vi "Unflatten.vi"(8 "error in (no error)":errorcluster, 11 "LCD Reader in":refnum<class "LCD Reader.lvclass">) -> (0 "error out":errorcluster, 3 "LCD Reader out":refnum<class "LCD Reader.lvclass">)   [LabVIEW 2012, in "LCD Reader.lvclass"]
uses:
  LCD Reader.lvclass
  Reader/Reader.lvclass
  LCD Reader.lvclass/LCD Reader.ctl
  Global/File Locations.vi
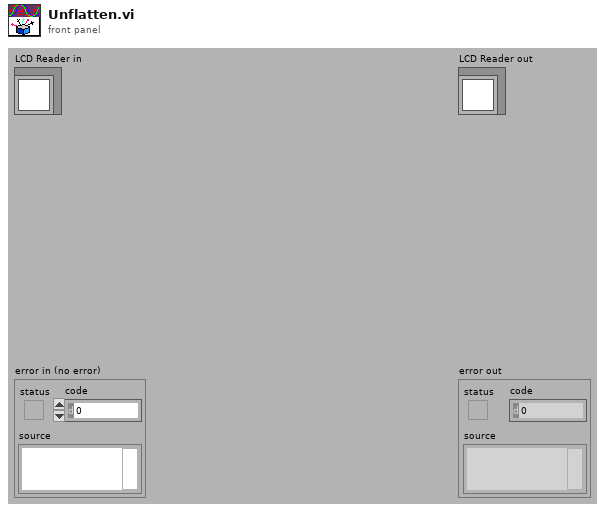
[diagram p1: front panel]
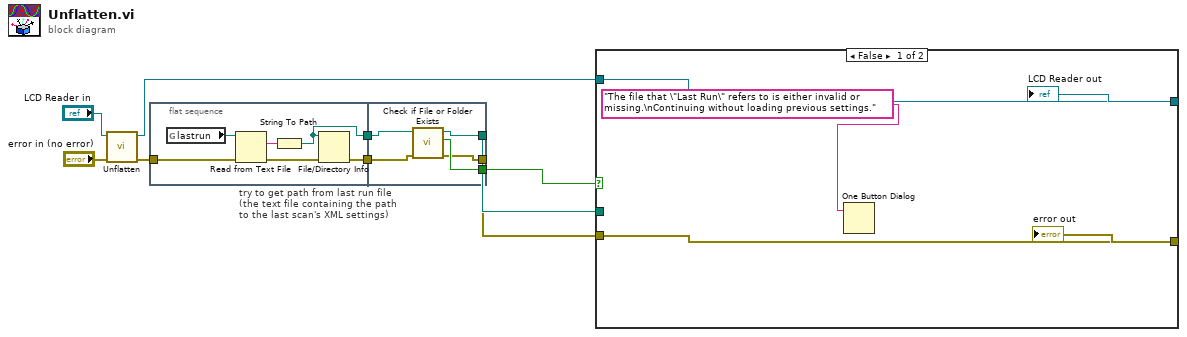
[diagram p0: block diagram]
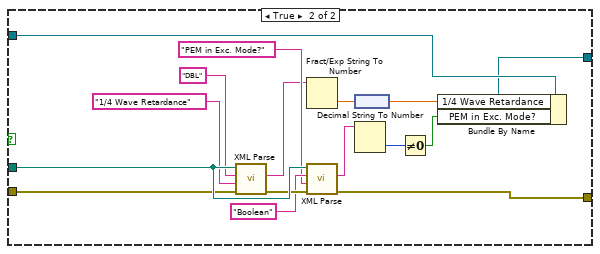
[diagram p2: hidden frame]
diagram:
  n1 = call-parent "Unflatten.vi"("error in (no error)"="error in (no error)", "Reader in"="LCD Reader in") -> ("error out"=w7:errorcluster, "Reader out"=w11:refnum<class "LCD Reader.lvclass">)  [unwired: 8 in]
  n2 = flat-sequence "try to get path from last run file\n(the text file containing the path\nto the last scan's XML settings)" {
    tunnel: w7 -> [w12]
    tunnel: [w17] -> w3
    tunnel: [w13] -> w2
    tunnel: [w20] -> w5
    tunnel: [w22] -> w6
    tunnel: w3 -> [w18]
    tunnel: w2 -> [w19]
    tunnel: [w21] -> w1
    frame #0 {
      n3 = global read "File Locations.vi" "lastrun"() -> (w15:path)
      n4 = Read from Text File(file (use dialog)=w15, error in=w12) -> (text=w16:string, error out=w14:errorcluster)  [unwired: 4 out]
      n5 = String To Path(string=w16) -> (path=w17:path)
      n6 = File/Directory Info(path=w17, error in=w14) -> (error out=w13:errorcluster)  [unwired: 6 out]
    }
    frame #1 {
      n7 = call <vilib>:"Check if File or Folder Exists.vi"("error in (no error)"=w19, "path"=w18) -> ("error out"=w20:errorcluster, "file or folder exists?"=w21:bool, "dup path"=w22:path)  [unwired: 7 in]
    }
  }
  n8 = case shown="False" w1 {
    tunnel: w11 -> [w25 w41]
    tunnel: [w25 w40] -> w8
    tunnel: w6 -> [_ w39]
    tunnel: w5 -> [w24 w38]
    tunnel: [w24 w36] -> w4
    frame False {
      n9 = One Button Dialog(message="The file that \"Last Run\" refers to is either invalid or missing.\nContinuing without loading previous settings.") -> ()  [unwired: 1 in, 1 out]
    }
    frame True {
      n10 = call "XML Parse.vi"("error in (no error)"=w38, "Name String"="1/4 Wave Retardance", "Type String"="DBL", "Path"=w39) -> ("error out"=w37:errorcluster, "String Out"=w31:string)  [unwired: 6 in]
      n11 = Fract/Exp String To Number(string=w31) -> (number=w30:dbl)  [unwired: 3 in, 1 out]
      n12 = call "XML Parse.vi"("error in (no error)"=w37, "Name String"="PEM in Exc. Mode?", "Type String"="Boolean", "Path"=w39) -> ("error out"=w36:errorcluster, "String Out"=w28:string)  [unwired: 6 in]
      n13 = node(w30) -> (w29:dbl[unit])
      n14 = Decimal String To Number(string=w28) -> (number=w27:i32)  [unwired: 2 in, 1 out]
      n15 = Not Equal To 0?(x=w27) -> (x != 0?=w26:bool)
      n16 = Bundle By Name(cluster=w41, "1/4 Wave Retardance"=w29, "PEM in Exc. Mode?"=w26) -> (w40:refnum<class "LCD Reader.lvclass">)
    }
  }
  "error out" <- w4
  "LCD Reader out" <- w8
